vi "Mutex Try Lock.vi"(8 "error in (no error)":errorcluster, 11 "Mutex in":T1) -> (0 "error out":errorcluster, 2 "lock success?":bool, 3 "Mutex out":T1)   [LabVIEW 2016, in "Linux RT IPC.POSIX Threads.lvlib" / "Mutex.lvclass"]
doc: "Calls pthread_mutex_trylock() on the pthread mutex object encapsulated by Mutex.\n\nThis VI attempts to lock the provided mutex. If the mutex is already locked, this VI will return and indicate that it was not successful. Otherwise, the mutex will be locked and this VI will return and indicate it was successful.\n\nRefer to online POSIX documentation for more information."
uses:
  Mutex.lvclass
  Controls/reference.ctl
  C:/Git/SourceTree/LinuxRT-IPC/Source/POSIX Threads/Classes/POSIX Thread Object/POSIX Thread Object.lvclass
  POSIX Thread Object/POSIX Thread Object.lvclass/POSIX Thread Object.ctl
  POSIX Thread Object/Private VIs/libpthread path.vi
  POSIX Thread Object/Private VIs/get pthread error.vi
  POSIX Thread Object/POSIX Thread Object.lvclass
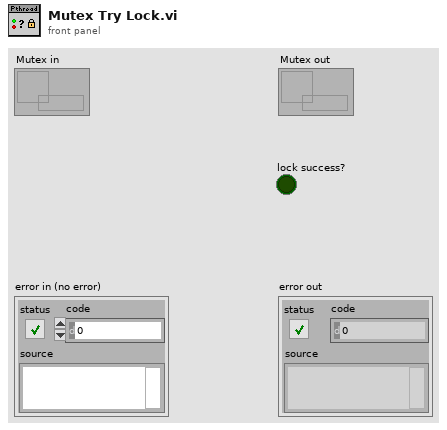
[diagram p1: front panel]
types:
  T1 = typedef "Linux RT IPC.POSIX Threads.lvlib/Mutex.lvclass/reference.ctl" = refnum<data-value>
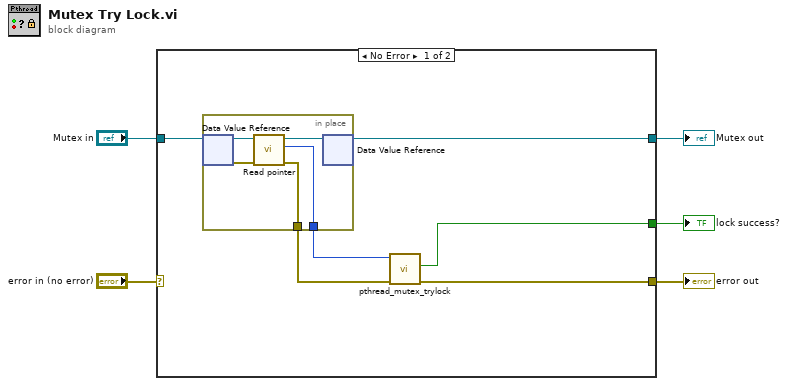
[diagram p0: block diagram]
diagram:
  n1 = case shown="No Error" "error in (no error)" {
    selector: "error in (no error)" -> [_ w18]
    tunnel: [w11 w18] -> w4
    tunnel: "Mutex in" -> [w9 w17]
    tunnel: [w8 w17] -> w2
    tunnel: [w10 _] -> w1
    frame No Error {
      n2 = in-place {
        in-place-border: [w13] -> w7
        in-place-border: [w12] -> w6
        n3 = in-place-dvr #1(w9) -> (w16:refnum<class "Mutex.lvclass">, w14:errorcluster)
        n4 = call "Read pointer.vi"("error in (no error)"=w14, "POSIX Thread Object in"=w16) -> ("error out"=w13:errorcluster, "pointer"=w12:u64, "POSIX Thread Object out"=w15:refnum<class "Mutex.lvclass">)  [unwired: 7 in]
        n5 = in-place-dvr #1(w15) -> (w8:T1)  [unwired: 1 out]
      }
      n6 = call "pthread_mutex_trylock.vi"("error in (no error)"=w7, "mutex ptr in"=w6) -> ("error out"=w11:errorcluster, "lock success?"=w10:bool)  [unwired: 7 in, 1 out]
    }
    frame Error {
    }
  }
  "Mutex out" <- w2
  "error out" <- w4
  "lock success?" <- w1
